vi "extractTags.vi"(8 "error in (no error)":errorcluster, 11 "tags":variant) -> (0 "error out":errorcluster, 1 "Setup":i32, 2 "Norm":i32, 3 "Test":i32, 4 "level":i32, 5 "isTest?":bool, 6 "img":i32)   [LabVIEW 2013, in "TreeRepresentation.lvlib"]
doc: "Zuordnung der Tags zu den dazugehörigen Daten-Objekten"
uses:
  lib/TreeRepresentation.lvlib
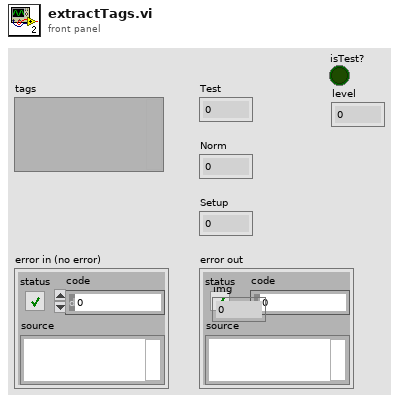
[diagram p1: front panel]
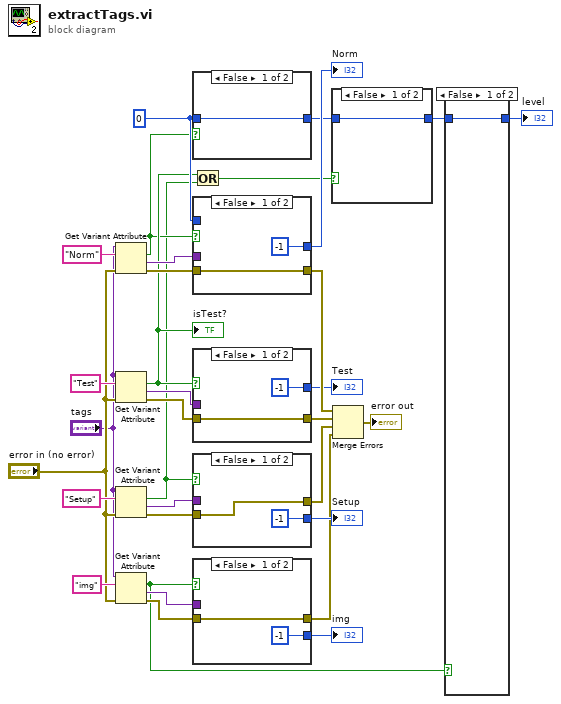
[diagram p0: block diagram]
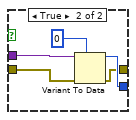
[diagram p2: hidden frame]
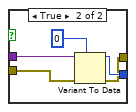
[diagram p3: hidden frame]
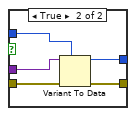
[diagram p4: hidden frame]
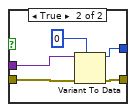
[diagram p5: hidden frame]
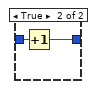
[diagram p6: hidden frame]
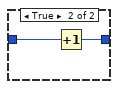
[diagram p7: hidden frame]
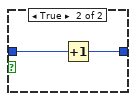
[diagram p8: hidden frame]
diagram:
  w16 = 0
  n1 = Get Variant Attribute(Variant="tags", name="Norm", error in="error in (no error)") -> (found=w3:bool, value=w18:variant, error out=w20:errorcluster)  [unwired: 1 in, 1 out]
  n2 = Get Variant Attribute(Variant="tags", name="Test", error in="error in (no error)") -> (found=w4:bool, value=w25:variant, error out=w26:errorcluster)  [unwired: 1 in, 1 out]
  "isTest?" <- w4
  n3 = Get Variant Attribute(Variant="tags", name="Setup", error in="error in (no error)") -> (found=w2:bool, value=w22:variant, error out=w21:errorcluster)  [unwired: 1 in, 1 out]
  n4 = Get Variant Attribute(Variant="tags", name="img", error in="error in (no error)") -> (found=w1:bool, value=w11:variant, error out=w12:errorcluster)  [unwired: 1 in, 1 out]
  n5 = case shown="False" w3 {
    tunnel: w16 -> [w33 w35]
    tunnel: [w33 w34] -> w15
    frame False {
    }
    frame True {
      n6 = Increment(x=w35) -> (x+1=w34:i32)
    }
  }
  n7 = Or(x=w4, y=w2) -> (x .or. y?=w6:bool)
  n8 = case shown="False" w3 {
    tunnel: [w36 w42] -> w28
    tunnel: w20 -> [w36 w41]
    tunnel: [-1 w40] -> w19
    tunnel: w18 -> [_ w39]
    tunnel: w16 -> [_ w38]
    frame False {
    }
    frame True {
      n9 = Variant To Data(error in=w41, type=w38, Variant=w39) -> (data=w40:i32, error out=w42:errorcluster)
    }
  }
  "Norm" <- w19
  n10 = case shown="False" w4 {
    tunnel: [w43 w49] -> w29
    tunnel: [-1 w48] -> w27
    tunnel: w26 -> [w43 w47]
    tunnel: w25 -> [_ w45]
    frame False {
    }
    frame True {
      n11 = Variant To Data(error in=w47, type=0, Variant=w45) -> (data=w48:i32, error out=w49:errorcluster)
    }
  }
  "Test" <- w27
  n12 = case shown="False" w2 {
    tunnel: [-1 w56] -> w31
    tunnel: [w50 w55] -> w30
    tunnel: w22 -> [_ w54]
    tunnel: w21 -> [w50 w52]
    frame False {
    }
    frame True {
      n13 = Variant To Data(error in=w52, type=0, Variant=w54) -> (data=w56:i32, error out=w55:errorcluster)
    }
  }
  "Setup" <- w31
  n14 = case shown="False" w1 {
    tunnel: w12 -> [w58 w63]
    tunnel: w11 -> [_ w61]
    tunnel: [-1 w60] -> w9
    tunnel: [w58 w59] -> w7
    frame False {
    }
    frame True {
      n15 = Variant To Data(error in=w63, type=0, Variant=w61) -> (data=w60:i32, error out=w59:errorcluster)
    }
  }
  "img" <- w9
  n16 = case shown="False" w6 {
    tunnel: w15 -> [w64 w66]
    tunnel: [w64 w65] -> w14
    frame False {
    }
    frame True {
      n17 = Increment(x=w66) -> (x+1=w65:i32)
    }
  }
  n18 = Merge Errors(w28, w29, w30, w7) -> (→"error out":errorcluster)
  n19 = case shown="False" w1 {
    tunnel: w14 -> [w67 w69]
    tunnel: [w67 w68] -> w13
    frame False {
    }
    frame True {
      n20 = Increment(x=w69) -> (x+1=w68:i32)
    }
  }
  "level" <- w13
